vi "ProcessTachometers.vi"(8 "error in (no error)":errorcluster, 9 "map":T2, 10 "Waveform":waveform(sgl), 11 "virtual channel in":T3) -> (0 "error out":errorcluster, 1 "map out":T2, 2 "pulse positions":T1, 3 "virtual channel out":T3)   [LabVIEW 2017, in "CmsVirtualChannel.lvlib"]
uses:
  <vilib>/addons/InsightCM/Devices/Shared/Cms/CmsVirtualChannel/CmsVirtualChannel.lvlib
  <vilib>/addons/PointValueMap/controls/PointMap.ctl
  <vilib>/addons/InsightCM/Devices/Shared/Cms/CmsVirtualChannel/controls/VirtualChannel.ctl
  <vilib>/addons/InsightCM/Utilities/Analysis/Shared/controls/PulsePositions.ctl
  <vilib>/addons/InsightCM/Devices/Shared/Cms/CmsVirtualChannel/controls/Tachometer.ctl
  <vilib>/addons/InsightCM/Utilities/Analysis/Vibration/controls/Tachometer.ctl
  <vilib>/addons/InsightCM/Utilities/Analysis/Vibration/controls/DigitalTachometer.ctl
  <vilib>/addons/InsightCM/Utilities/Analysis/Vibration/VibrationAnalysisFunctions.lvlib
  <vilib>/addons/InsightCM/Utilities/Analysis/Shared/AnalysisHelper.lvlib
  <vilib>/addons/PointValueMap/PointValueMap.lvlib
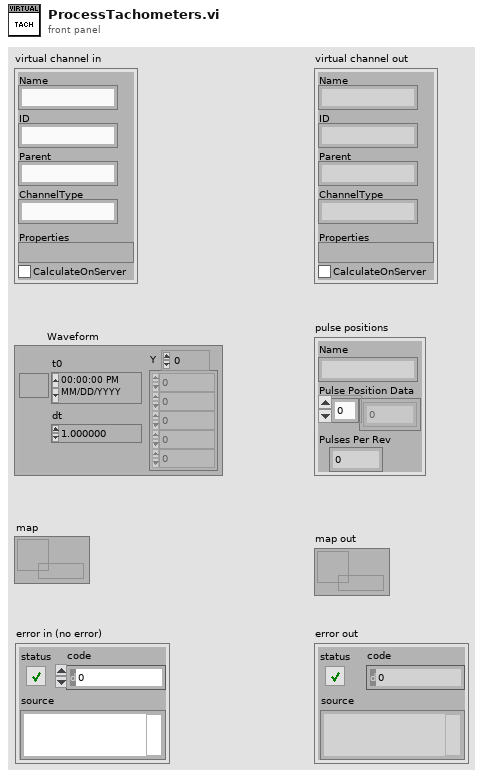
[diagram p1: front panel]
types:
  T1 = typedef "AnalysisHelper.lvlib/PulsePositions.ctl" = cluster{"Name":string, "Pulse Position Data":dbl[], "Pulses Per Rev":i32}
  T2 = typedef "PointValueMap.lvlib/PointMap.ctl" = refnum<data-value>
  T3 = typedef "CmsVirtualChannel.lvlib/VirtualChannel.ctl" = cluster{"Name":string, "ID":string, "Parent":string, "ChannelType":string, "Properties":variant, "CalculateOnServer":bool}
  T4 = typedef "CmsVirtualChannel.lvlib/Tachometer.ctl" = cluster{"Tachometer Slope":string, "Pulses Per Rev":i32, "Tachometer Threshold":dbl, "Tachometer Hysteresis":dbl, "Sensitivity":dbl, "Type":string, "Tach State":T5, "Settling Time":dbl}
  T5 = typedef "VibrationAnalysisFunctions.lvlib/Tachometer.ctl" = cluster{"Reset":bool, "analog tach state":cluster{"last value":dbl, "edge state":cluster{"processed data":dbl, "buffer data":dbl[]}}, "digital tach state in":T6, "speed state":cluster{"state":enum16{"0 Pulses", "1 Pulse", "2+ Pulses"}, "last pulse position":dbl, "RPM":dbl, "Empty Blocks":i32}}
  T6 = typedef "VibrationAnalysisFunctions.lvlib/DigitalTachometer.ctl" = cluster{dbl[], i32, "not enough pulses?":bool, "pulse buffer out":dbl[], i32, "final state":dbl[], "duration":dbl, "reset":bool, "overflow state":cluster{"low speed state":cluster{dbl, ext}, "counter state":cluster{"counter task type":enum16{"period measurement", "event counting"}, "t":dbl, "t":dbl}}, "OS Clk Start":dbl}
  T7 = typedef "OAT Position Info.ctl" = cluster{"positions [s]":dbl[], "samples/rev":dbl}
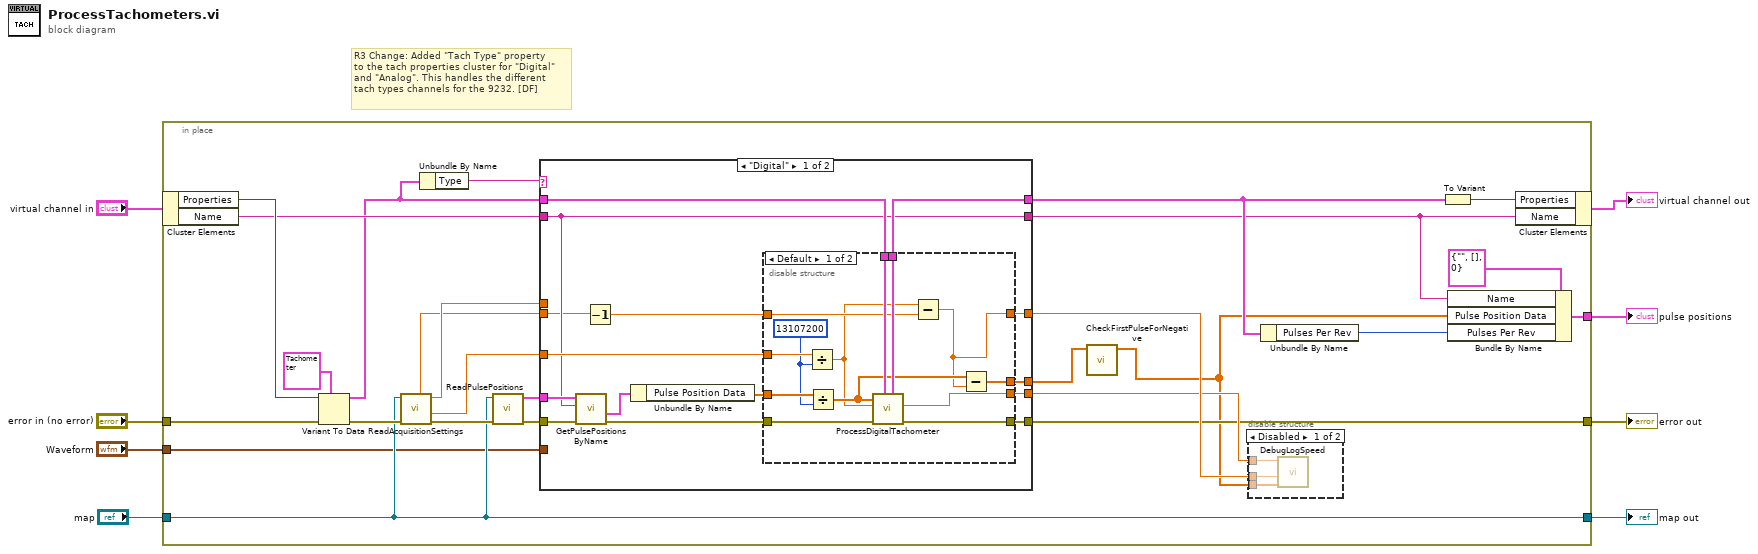
[diagram p0: block diagram]
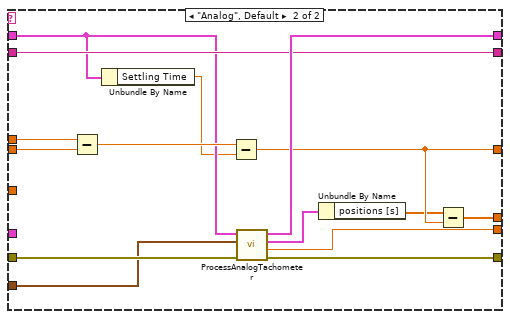
[diagram p4: hidden frame]
diagram:
  # "R3 Change: Added \"Tach Type\" property\nto the tach properties cluster for \"Digital\"\nand \"Analog\". This handles the different\ntach types channels for the 9232. [DF]"
  n1 = in-place {
    in-place-border: [w15] -> w8
    in-place-border: "map" -> [w14]
    in-place-border: "error in (no error)" -> [w29]
    in-place-border: [w14] -> w3
    in-place-border: [w16] -> w2
    in-place-border: "Waveform" -> [w9]
    n2 = in-place-cluster #1("virtual channel in") -> ("Properties"=w31:variant, "Name"=w23:string)
    n3 = Variant To Data(error in=w29, type=T4 {"Tachometer Slope"="", "Pulses Per Rev"=0, "Tachometer Threshold"=0.0, "Tachometer Hysteresis"=0.0, "Sensitivity"=0.0, "Type"="", "Tach State"={"Reset"=FALSE, "analog tach state"={"last value"=0.0, "edge state"={"processed data"=0.0, "buffer data"=[]}}, "digital tach state in"={[], 0, "not enough pulses?"=FALSE, "pulse buffer out"=[], 0, "final state"=[], "duration"=0.0, "reset"=FALSE, "overflow state"={"low speed state"={0.0, 0.0}, "counter state"={"counter task type"=enum."period measurement", "t"=0.0, "t"=0.0}}, "OS Clk Start"=0.0}, "speed state"={"state"=enum."0 Pulses", "last pulse position"=0.0, "RPM"=0.0, "Empty Blocks"=0}}, "Settling Time"=0.0} ("Tachometer"), Variant=w31) -> (data=w11:T4, error out=w26:errorcluster)
    n4 = call <vilib>:"ReadAcquisitionSettings.vi"("error in (no error)"=w26, "Map"=w14) -> ("error out"=w22:errorcluster, "OSClkStart"=w27:dbl, "Running Acquisition Length"=w28:dbl, "Block Size (s)"=w25:dbl)  [unwired: 4 in, 2 out]
    n5 = Unbundle By Name(w11) -> ("Type"=w10:string)
    n6 = call <vilib>:"ReadPulsePositions.vi"("error in (no error)"=w22, "Map"=w14) -> ("error out"=w21:errorcluster, "pulse positions array"=w20:T1[])  [unwired: 7 in, 1 out]
    n7 = case shown="\"Digital\"" w10 {
      tunnel: w21 -> [w45 w83]
      tunnel: [w52 w82] -> w15
      tunnel: [w51 w81] -> w32
      tunnel: w28 -> [_ w77]
      tunnel: [w47 w74] -> w33
      tunnel: w27 -> [w50 _]
      tunnel: w23 -> [w42 w78]
      tunnel: [w49 w80] -> w24
      tunnel: w11 -> [w48 w71]
      tunnel: [w46 w72] -> w13
      tunnel: [w42 w78] -> w18
      tunnel: w25 -> [w39 w76]
      tunnel: w20 -> [w43 _]
      tunnel: w9 -> [_ w69]
      frame "Digital" {
        n8 = call <vilib>:"GetPulsePositionsByName.vi"("error in (no error)"=w45, "Channel Name"=w42, "Pulse Positions Array"=w43) -> ("error out"=w44:errorcluster, "Pulse Positions"=w41:T1)  [unwired: 5 in, 2 out]
        n9 = Decrement(x=w39) -> (x-1=w38:dbl)
        n10 = Unbundle By Name(w41) -> ("Pulse Position Data"=w40:dbl[])
        n11 = disable-structure shown="Default" {
          disable-tunnel: [w65 w66] -> w52
          disable-tunnel: [w64 _] -> w51
          disable-tunnel: w50 -> [w63 _]
          disable-tunnel: [w62 w67] -> w49
          disable-tunnel: w48 -> [w61 w67]
          disable-tunnel: [w53 _] -> w47
          disable-tunnel: [w60 w68] -> w46
          disable-tunnel: w44 -> [w59 w66]
          disable-tunnel: w40 -> [w58 w68]
          disable-tunnel: w38 -> [w55 _]
          frame condition #0 (active) {
            w57 = u32 13107200 ("y")
            n12 = Divide(x=w63, y=w57) -> (x/y=w54:dbl)
            n13 = Divide(x=w58, y=w57) -> (x/y=w56:dbl[])
            n14 = call <vilib>:"ProcessDigitalTachometer.vi"("Tachometer in"=w61, "error in (no error)"=w59, "OS Clk Start"=w54, "pulses"=w56) -> ("error out"=w65:errorcluster, "Instant RPM"=w64:dbl, "Tachometer out"=w62:T4)  [unwired: 4 in, 1 out]
            n15 = Subtract(x=w54, y=w55) -> (x-y=w53:dbl)
            n16 = Subtract(x=w56, y=w53) -> (x-y=w60:dbl[])
          }
          frame condition #1 {
          }
        }
      }
      frame "Analog", Default {
        n17 = Subtract(x=w77, y=w76) -> (x-y=w75:dbl)
        n18 = Unbundle By Name(w71) -> ("Settling Time"=w70:dbl)
        n19 = Subtract(x=w75, y=w70) -> (x-y=w74:dbl)
        n20 = call <vilib>:"ProcessAnalogTachometer.vi"("error in (no error)"=w83, "waveform"=w69, "tachometer"=w71) -> ("error out"=w82:errorcluster, "instanteous speed (RPM)"=w81:dbl, "speed position info"=w79:T7, "tachometer out"=w80:T4)  [unwired: 5 in]
        n21 = Unbundle By Name(w79) -> ("positions [s]"=w73:dbl[])
        n22 = Subtract(x=w73, y=w74) -> (x-y=w72:dbl[])
      }
    }
    n23 = call <vilib>:"CheckFirstPulseForNegative.vi"("pulses in"=w13) -> ("pulses out"=w12:dbl[])  [unwired: 10 in]
    n24 = disable-structure shown="Disabled" {
      disable-tunnel: w32 -> [w35 _]
      disable-tunnel: w33 -> [w36 _]
      disable-tunnel: w12 -> [w37 _]
      frame Disabled {
        n25 = call <vilib>:"DebugLogSpeed.vi"("positions [s]"=w37, "t0"=w36, "Instant RPM"=w35) -> ()  [unwired: 9 in]
      }
      frame Enabled {
      }
    }
    n26 = Unbundle By Name(w24) -> ("Pulses Per Rev"=w17:i32)
    n27 = To Variant(anything=w24) -> (Variant=w30:variant)
    n28 = Bundle By Name(cluster=T1 {"Name"="", "Pulse Position Data"=[], "Pulses Per Rev"=0} ("Pulse Positions"), "Name"=w18, "Pulse Position Data"=w12, "Pulses Per Rev"=w17) -> (w16:T1)
    n29 = in-place-cluster #1("Properties"=w30, "Name"=w18) -> (→"virtual channel out":T3)
  }
  "error out" <- w8
  "map out" <- w3
  "pulse positions" <- w2
